vi "FRCts20_Backend_TempDirGen.vi"(6 "error in (no error) 2":errorcluster, 8 "Temporary File Extension (tmp)":string="tmp") -> (0 "error out 2":errorcluster, 2 "Unique Temporary File Path":path)   [LabVIEW 2014, in "FRCts20_Backend_Engine_Deprecated.lvlib"]
uses:
  FRCts20_Backend_Engine_Deprecated.lvlib
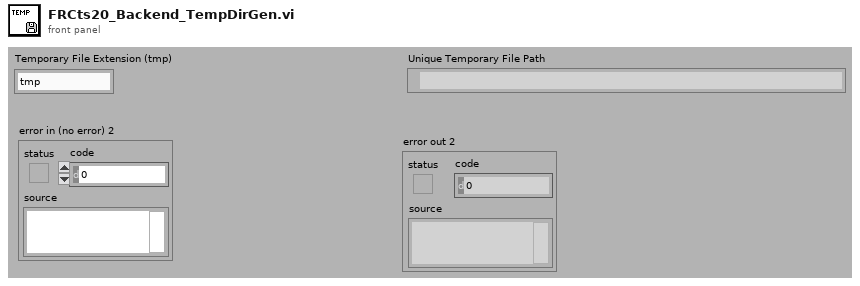
[diagram p1: front panel]
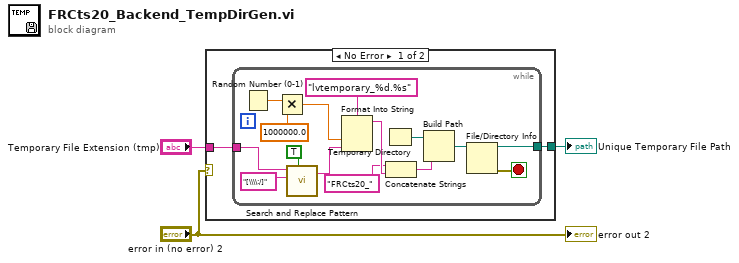
[diagram p0: block diagram]
diagram:
  n1 = case shown="No Error" "error in (no error) 2" {
    tunnel: "Temporary File Extension (tmp)" -> [w5 _]
    tunnel: [w4 _] -> w3
    frame No Error {
      n2 = while {
        tunnel: w5 -> [w12]
        tunnel: [w13] -> w4
        stop <- w14 stop-if-true
        n3 = Random Number (0-1)() -> (number: 0 to 1=w20:dbl)
        n4 = Multiply(x=w20, y=1000000.0) -> (x*y=w17:dbl)
        n5 = call <vilib>:"Search and Replace Pattern.vi"("string"=w12, "regular expression (\"\")"="[\\\\:/]" ("regular expression (\"\")"), "replace all? (F)"=TRUE) -> ("result string"=w11:string)  [unwired: 1 in, 2 out]
        n6 = Format Into String(format string="lvtemporary_%d.%s", w17, w11) -> (resulting string=w8:string)  [unwired: 2 in, 1 out]
        n7 = Temporary Directory() -> (w16:path)
        n8 = Concatenate Strings("FRCts20_" ("string"), w8) -> (w7:string)
        n9 = Build Path(base path=w16, name or relative path=w7) -> (appended path=w15:path)
        n10 = File/Directory Info(path=w15) -> (path out=w13:path, error out=w14:errorcluster)  [unwired: 1 in, 5 out]
      }
    }
    frame Error {
    }
  }
  "Unique Temporary File Path" <- w3
  "error out 2" <- "error in (no error) 2"
